vi "Parse updateNewMessage.vi"(8 "error in (no error)":errorcluster, 11 "JSON (UTF-8) String":string) -> (0 "error out":errorcluster, 2 "Telegram State":T1, 3 "Message":variant)   [LabVIEW 2015, in "JSON Library.lvlib"]
doc: "Created IvanLis by LabVIEW Portal\nProfile: http://labviewportal.org/memberlist.php?mode=viewprofile&u=987\neMail: IvanLisanov@gMail.com\nTelegram: https://t.me/IvanLis"
uses:
  JSON Library.lvlib
  Telegram Library/TypeDef/Telegram State.ctl
  TypeDef/Message Text.ctl
  Telegram Library/Telegram Library.lvlib
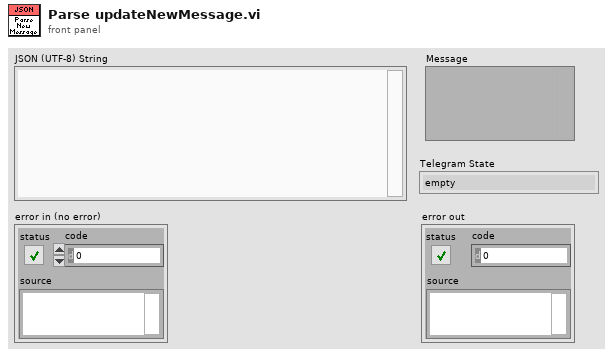
[diagram p1: front panel]
types:
  T1 = typedef "Telegram Library.lvlib/Telegram State.ctl" = enum16{"empty", "ok", "authorizationStateClosed", "authorizationStateWaitTdlibParameters", "authorizationStateWaitEncryptionKey", "authorizationStateWaitPhoneNumber", "authorizationStateWaitCode", "connectionStateWaitingForNetwork", "connectionStateConnectingToProxy", "connectionStateUpdating", "connectionStateConnecting", "connectionStateReady", "updateUser_user", "updateNewChat_chat", "updateNewMessage_Text", "updateChatLastMessage_Text", "updateDeleteMessages", "updateChatPosition", "ChatHistoryMessages_Text"}
  T2 = typedef "JSON Library.lvlib/Message Text.ctl" = cluster{"@type":string, "id":i64, "sender_id":cluster{"@type":string, "user_id":i64}, "chat_id":i64, "date":i64, "content":cluster{"@type":string, "text":cluster{"@type":string, "text":string}}}
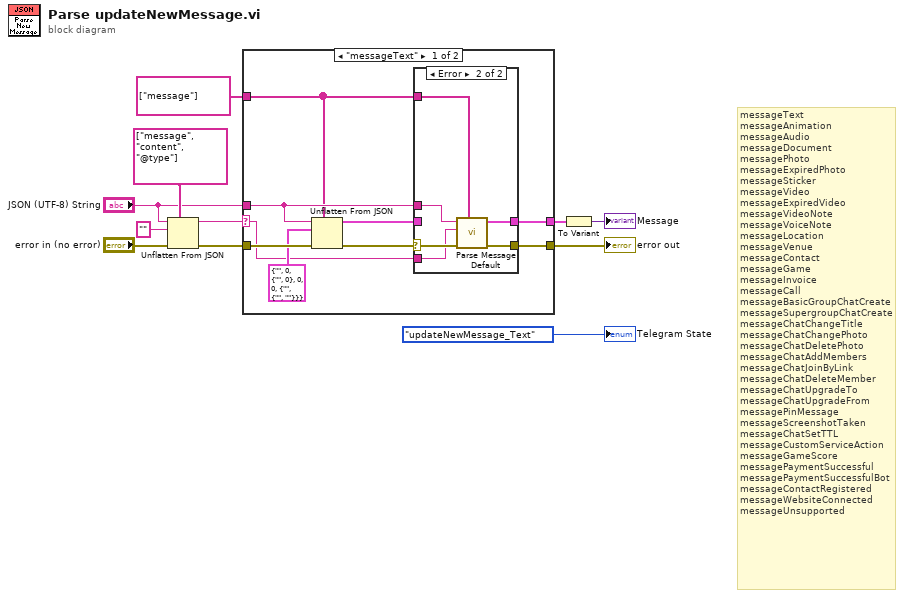
[diagram p0: block diagram]
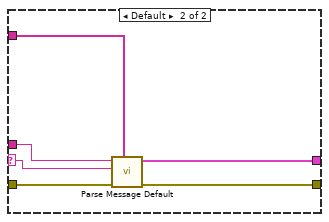
[diagram p3: hidden frame]
diagram:
  # "messageText\nmessageAnimation\nmessageAudio\nmessageDocument\nmessagePhoto\nmessageExpiredPhoto\nmessageSticker\nmessageVideo\nmessageExpiredVideo\nmessageVideoNote\nmessageVoiceNote\nmessageLocation\nmessageVenue\nmessageContact\nmessageGame\nmessageInvoice\nmessageCall\nmessageBasicGroupChatCreate\nmessageSupergroupChatCreate\nmessageChatChangeTitle\nmessageChatChangePhoto\nmessageChatDeletePhoto\nmessageChatAddMembers\nmessageChatJoinByLink\nmessageChatDeleteMember\nmessageChatUpgradeTo\nmessageChatUpgradeFrom\nmessagePinMessage\nmessageScreenshotTaken\nmessageChatSetTTL\nmessageCustomServiceAction\nmessageGameScore\nmessagePaymentSuccessful\nmessagePaymentSuccessfulBot\nmessageContactRegistered\nmessageWebsiteConnected\nmessageUnsupported"
  n1 = Unflatten From JSON(path=string[] ["message", "content", "@type"], JSON string="JSON (UTF-8) String", type and defaults="", error in (no error)="error in (no error)") -> (value=w9:string, error out=w6:errorcluster)  [unwired: 3 in]
  n2 = case shown="\"messageText\"" w9 {
    selector: w9 -> [w13 w30]
    tunnel: w6 -> [w20 w34]
    tunnel: [w15 w32] -> w3
    tunnel: [w17 w33] -> w10
    tunnel: "JSON (UTF-8) String" -> [w14 w31]
    tunnel: string[] ["message"] ("path") -> [w12 w29]
    frame "messageText" {
      n3 = Unflatten From JSON(path=w12, JSON string=w14, type and defaults=T2 {"@type"="", "id"=0, "sender_id"={"@type"="", "user_id"=0}, "chat_id"=0, "date"=0, "content"={"@type"="", "text"={"@type"="", "text"=""}}} ("New Message Text"), error in (no error)=w20) -> (value=w16:T2, error out=w18:errorcluster)  [unwired: 3 in]
      n4 = case shown="Error" w18 {
        selector: w18 -> [w21 w28]
        tunnel: w16 -> [w22 _]
        tunnel: [w22 w26] -> w17
        tunnel: [w21 w27] -> w15
        tunnel: w14 -> [_ w25]
        tunnel: w13 -> [_ w24]
        tunnel: w12 -> [_ w23]
        frame No Error {
        }
        frame Error {
          n5 = call "Parse Message Default.vi"("path"=w23, "error in (no error)"=w28, "content.@type"=w24, "JSON (UTF-8) String"=w25) -> ("error out"=w27:errorcluster, "New Message Text"=w26:T2)  [unwired: 6 in]
        }
      }
    }
    frame Default {
      n6 = call "Parse Message Default.vi"("path"=w29, "error in (no error)"=w34, "content.@type"=w30, "JSON (UTF-8) String"=w31) -> ("error out"=w32:errorcluster, "New Message Text"=w33:T2)  [unwired: 6 in]
    }
  }
  "error out" <- w3
  n7 = To Variant(anything=w10) -> (Variant=→"Message":variant)
  "Telegram State" <- Telegram_State."updateNewMessage_Text" ("Telegram State")
